vi "Test Micron sm.vi"() -> ()   [LabVIEW 2024]
uses:
  Micron Optics sm130/Micron Optics sm130.lvlib
panel:
  out "Trig type check":string
  in  "Trigger Stop Edge (0: Rising)":u16(ring) items=["Rising", "Falling", "NONE"]
  out "Waveform Graph 2":dbl[](graph)
  out "Peak Wavelengths (nm)":dbl[][](array[numeric])
  out "size(s)":i32[](array[numeric])
  out "Initial count":i32
  in  "milliseconds to wait":u32=1000
  out "Data serial number":u32[](array[numeric])
  out "Buffer count":i32[](array[numeric])
  in  "ID Query (True)":bool=TRUE
  in  "Send stop":bool
  out "Stop sent":bool
  out "elapsed time":u32
  out "Final count":i32
  in  "extra counts":i32=1000
  in  "Count progress":bool
  out "Array":bool[](array[boolean])
  in  "Enable Unbuffered Data (Enabled)":bool=TRUE
  out "Waveform Graph":dbl[](graph)
  in  "Channel (1: Channel 1)":i32(ring)=2 items=["Channel 1"=1, "Channel 2"=2, "Channel 3"=3, "Channel 4"=4]
  in  "Sensor Number (1)":i32=1
  out "Set Buffer Response":string
  out "Trig Response":string[](array[string])
  in  "Number of Acquisitions (100)":i32=100
  in  "Trigger Stop Condition (1:Edge Triggering)":u16(ring) items=["Number of Acquisitions", "Edge Triggering"]
  in  "Trigger Type (0:Untriggered)":u16(ring)=1 items=["Untriggered", "Software Triggered", "Hardware Triggered"]
  in  "VISA resource name":refnum<visa-resource-name>="TCPIP0::192.168.1.69::1852::SOCKET"
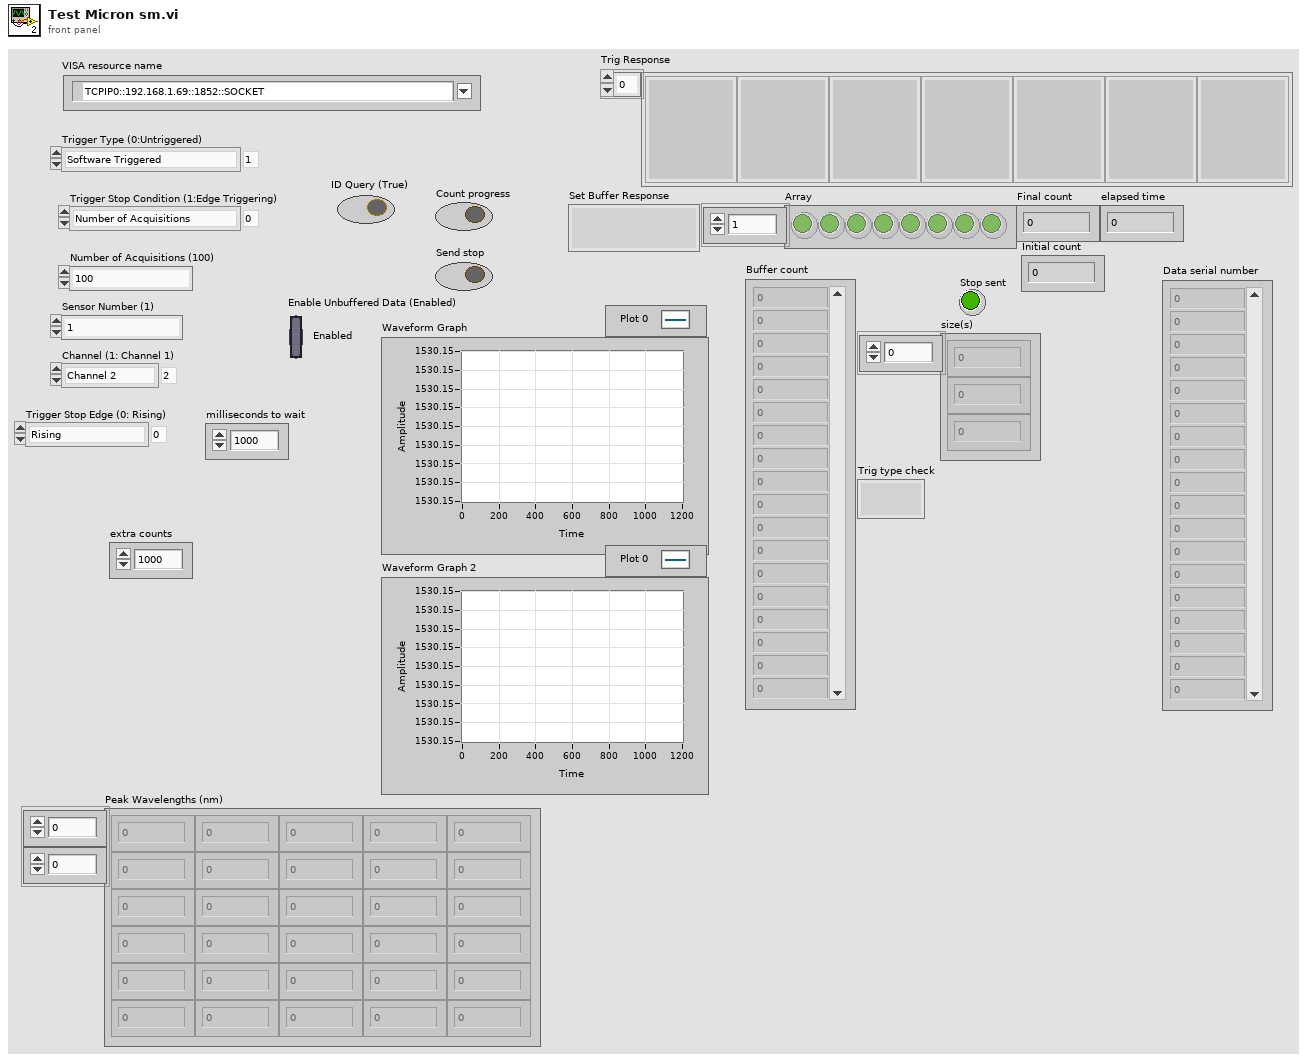
[diagram p1: front panel]
types:
  T1 = cluster{"Data Serial Number":u32, "Time Stamp":dbl, "Sub-Channel":u8}
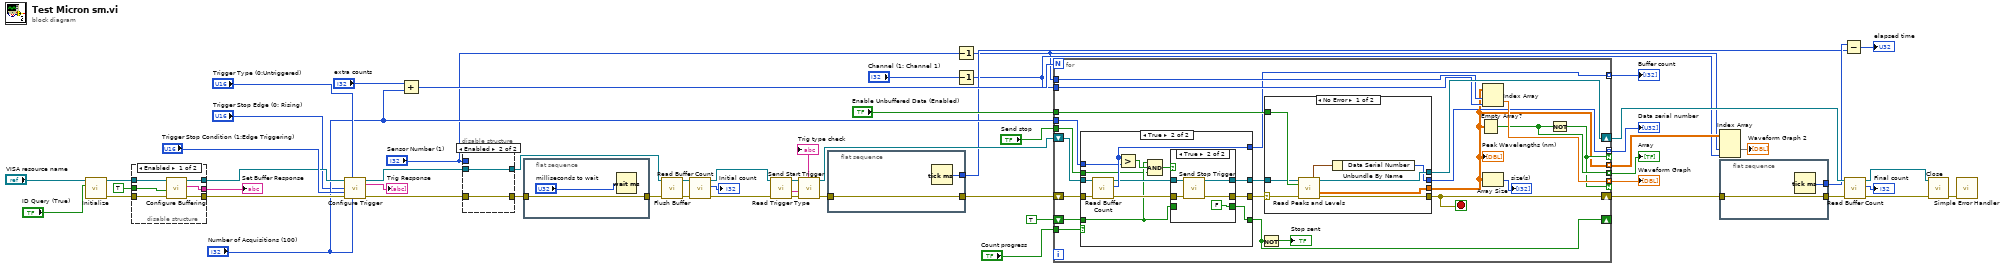
[diagram p0: block diagram]
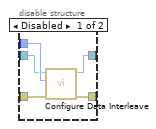
[diagram p2: hidden frame]
diagram:
  n1 = call "Initialize.vi"("ID Query (True)"="ID Query (True)", "VISA resource name"="VISA resource name") -> ("error out"=w48:errorcluster, "VISA resource name out"=w47:refnum<visa-resource-name>)  [unwired: 8 in]
  n2 = disable-structure shown="Enabled" {
    disable-tunnel: TRUE ("Enable Buffering (Enable)") -> [w61 _]
    disable-tunnel: [w60 _] -> w49
    disable-tunnel: w48 -> [w59 w63]
    disable-tunnel: w47 -> [w58 w62]
    disable-tunnel: [w57 w62] -> w46
    disable-tunnel: [w56 w63] -> w45
    frame Enabled {
      n3 = call "Configure Buffering.vi"("error in (no error)"=w59, "Enable Buffering (Enable)"=w61, "VISA resource name"=w58) -> ("error out"=w56:errorcluster, "Confirmation Response"=w60:string, "VISA resource name out"=w57:refnum<visa-resource-name>)  [unwired: 6 in]
    }
    frame Disabled {
    }
  }
  "Set Buffer Response" <- w49
  n4 = call "Configure Trigger.vi"("VISA resource name"=w46, "Trigger Type (0:Untriggered)"="Trigger Type (0:Untriggered)", "Trigger Stop Edge (0: Rising)"="Trigger Stop Edge (0: Rising)", "Trigger Stop Condition (1:Edge Triggering)"="Trigger Stop Condition (1:Edge Triggering)", "error in (no error)"=w45, "Number of Acquisitions (100)"="Number of Acquisitions (100)") -> ("VISA resource name out"=w41:refnum<visa-resource-name>, "Response"=→"Trig Response":string[], "error out"=w40:errorcluster)  [unwired: 7 in]
  n5 = Add(x="extra counts", y="Number of Acquisitions (100)") -> (x+y=w37:i32)
  n6 = disable-structure shown="Enabled" {
    disable-tunnel: "Sensor Number (1)" -> [w68 _]
    disable-tunnel: w41 -> [w67 w70]
    disable-tunnel: w40 -> [w66 w69]
    disable-tunnel: [w65 w69] -> w17
    disable-tunnel: [w64 w70] -> w13
    frame Disabled {
      n7 = call "Configure Data Interleave.vi"("error in (no error)"=w66, "Sensor Number (1)"=w68, "VISA resource name"=w67) -> ("error out"=w65:errorcluster, "VISA resource name out"=w64:refnum<visa-resource-name>)  [unwired: 7 in]
    }
    frame Enabled {
    }
  }
  n8 = flat-sequence {
    tunnel: w17 -> [w72]
    tunnel: [w72] -> w15
    frame #0 {
      n9 = Wait (ms)(milliseconds to wait="milliseconds to wait") -> ()  [unwired: 1 out]
    }
  }
  n10 = call "Flush Buffer.vi"("error in (no error)"=w15, "VISA resource name"=w13) -> ("error out"=w14:errorcluster, "VISA resource name out"=w12:refnum<visa-resource-name>)  [unwired: 8 in]
  n11 = call "Read Buffer Count.vi"("error in"=w14, "VISA resource name"=w12) -> ("error out"=w3:errorcluster, "count"=→"Initial count":i32, "VISA resource name out"=w5:refnum<visa-resource-name>)  [unwired: 6 in, 1 out]
  n12 = call "Read Trigger Type.vi"("error in"=w3, "VISA resource name"=w5) -> ("error out"=w2:errorcluster, "Confirmation Response"=→"Trig type check":string, "VISA resource name out"=w4:refnum<visa-resource-name>)  [unwired: 6 in, 1 out]
  n13 = call "Send Start Trigger.vi"("error in (no error)"=w2, "VISA resource name"=w4) -> ("error out"=w28:errorcluster, "VISA resource name out"=w39:refnum<visa-resource-name>)  [unwired: 8 in]
  n14 = flat-sequence {
    tunnel: w28 -> [w74]
    tunnel: [w74] -> w27
    tunnel: [w73] -> w23
    frame #0 {
      n15 = Tick Count (ms)() -> (millisecond timer value=w73:u32)
    }
  }
  n16 = Decrement(x="Sensor Number (1)") -> (x-1=w7:i32)
  n17 = Decrement(x="Channel (1: Channel 1)") -> (x-1=w10:i32)
  n18 = for {
    N: w37 -> [_]
    shift-right: [w95] -> w26
    shift-left: w27 -> [w89]
    shift-right: [w96] -> w34
    shift-left: w39 -> [w90]
    tunnel: w7 -> [w94]
    tunnel: w10 -> [w93]
    tunnel: [w92] -> w43 mode=indexing if=w77
    tunnel: "Enable Unbuffered Data (Enabled)" -> [w91]
    tunnel: [w86] -> w38 mode=indexing
    tunnel: [w84] -> w19 mode=indexing
    tunnel: "Count progress" -> [w85]
    tunnel: "Number of Acquisitions (100)" -> [w83]
    shift-right: [w81] -> _
    shift-left: TRUE -> [w82]
    tunnel: "Send stop" -> [w79]
    tunnel: [w78] -> w18 mode=indexing if=w77
    tunnel: [w75] -> w11 mode=indexing
    stop <- w95 stop-if-true
    n19 = case shown="True" w85 {
      tunnel: w90 -> [w98 w112]
      tunnel: w89 -> [w99 w111]
      tunnel: [w98 w105] -> w88
      tunnel: [w99 w103] -> w87
      tunnel: [_ w110] -> w84
      tunnel: w83 -> [_ w109]
      tunnel: w82 -> [w97 w102]
      tunnel: [w97 w101] -> w81
      tunnel: w79 -> [_ w100]
      frame False {
      }
      frame True {
        n20 = call "Read Buffer Count.vi"("error in"=w111, "VISA resource name"=w112) -> ("error out"=w104:errorcluster, "count"=w110:i32, "VISA resource name out"=w106:refnum<visa-resource-name>)  [unwired: 6 in, 1 out]
        n21 = Greater?(x=w110, y=w109) -> (0:w108:bool)
        n22 = Compound Arithmetic op=AND(w102, w108, w100) -> (w107:bool)
        n23 = case shown="True" w107 {
          tunnel: w106 -> [w115 w120]
          tunnel: [w115 w119] -> w105
          tunnel: w104 -> [w114 w118]
          tunnel: [w114 w117] -> w103
          tunnel: w102 -> [w113 _]
          tunnel: [w113 FALSE] -> w101
          frame False {
          }
          frame True {
            n24 = call "Send Stop Trigger.vi"("error in (no error)"=w118, "VISA resource name"=w120) -> ("error out"=w117:errorcluster, "VISA resource name out"=w119:refnum<visa-resource-name>)  [unwired: 8 in]
          }
        }
      }
    }
    n25 = Not(x=w81) -> (.not. x?=→"Stop sent":bool)
    n26 = case shown="No Error" w87 {
      selector: w87 -> [w123 w130]
      tunnel: [w128 w129] -> w96
      tunnel: [w127 w130] -> w95
      tunnel: [w126 _] -> w75
      tunnel: w91 -> [w125 _]
      tunnel: w88 -> [w124 w129]
      tunnel: [w121 _] -> w78
      frame No Error {
        n27 = call "Read Peaks and Levels.vi"("VISA resource name"=w124, "Enable Unbuffered Data (Enabled)"=w125, "error in (no error)"=w123) -> ("Data Status"=w122:T1, "VISA resource name out"=w128:refnum<visa-resource-name>, "Peak Wavelengths (nm)"=w126:dbl[][], "error out"=w127:errorcluster)  [unwired: 4 in, 5 out]
        n28 = Unbundle By Name(w122) -> ("Data Serial Number"=w121:u32)
      }
      frame Error {
      }
    }
    "Peak Wavelengths (nm)" <- w75
    n29 = Empty Array?(array=w75) -> (empty?=w86:bool)
    n30 = Index Array(array=w75, index (row)=w94, index (col)=w93) -> (element=w92:dbl)
    n31 = Array Size(array=w75) -> (size(s)=→"size(s)":i32[])
    n32 = Not(x=w86) -> (.not. x?=w77:bool)
  }
  "Waveform Graph" <- w43
  "Array" <- w38
  "Buffer count" <- w19
  "Data serial number" <- w18
  n33 = Index Array(array=w11, index (dim 1)=w7, index (dim 2)=w10) -> (element=→"Waveform Graph 2":dbl[])  [unwired: 1 in]
  n34 = flat-sequence {
    tunnel: w26 -> [w132]
    tunnel: [w132] -> w25
    tunnel: [w131] -> w24
    frame #0 {
      n35 = Tick Count (ms)() -> (millisecond timer value=w131:u32)
    }
  }
  n36 = Subtract(x=w24, y=w23) -> (x-y=→"elapsed time":u32)
  n37 = call "Read Buffer Count.vi"("error in"=w25, "VISA resource name"=w34) -> ("error out"=w35:errorcluster, "count"=→"Final count":i32, "VISA resource name out"=w33:refnum<visa-resource-name>)  [unwired: 6 in, 1 out]
  n38 = call "Close.vi"("error in (no error)"=w35, "VISA resource name"=w33) -> ("error out"=w53:errorcluster)  [unwired: 9 in]
  n39 = call <vilib>:"Simple Error Handler.vi"("error in (no error)"=w53) -> ()  [unwired: 4 in, 5 out]
